vi "Host Error log.vi"(6 "Operation":enum16{"Create", "Write", "Close", "Header"}(ring)=enum."Write", 8 "error in":errorcluster, 11 "Enable":bool) -> (0 "error out":errorcluster, 2 "Error":string[][](array[string]))   [LabVIEW 2021]
uses:
  <vilib>/Utility/sysdir.llb/System Directory Type.ctl
  Main Engine/Controls/Main Engine Q Option.ctl
panel:
  in  "error in 2":errorcluster={"status"=TRUE, "code"=1, "source"="Dequeue Element in Host Error log.vi->MATSYA GUI.vi"}
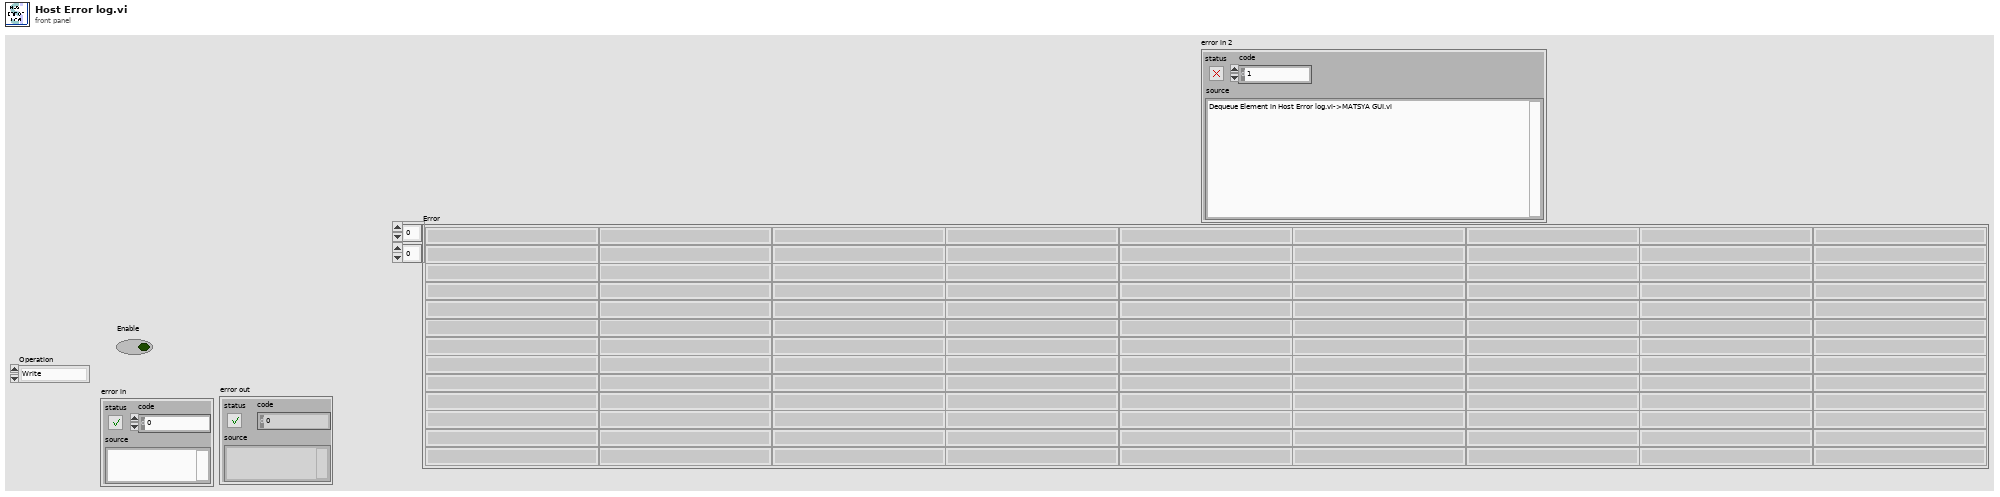
[diagram p1: front panel]
types:
  T1 = enum16{"open", "replace", "create", "open or create", "replace or create", "replace or create with confirmation"}
  T2 = typedef "Main Engine Q Option.ctl" = enum16{"Init", "Get"}
  T3 = typedef "System Directory Type.ctl" = i32
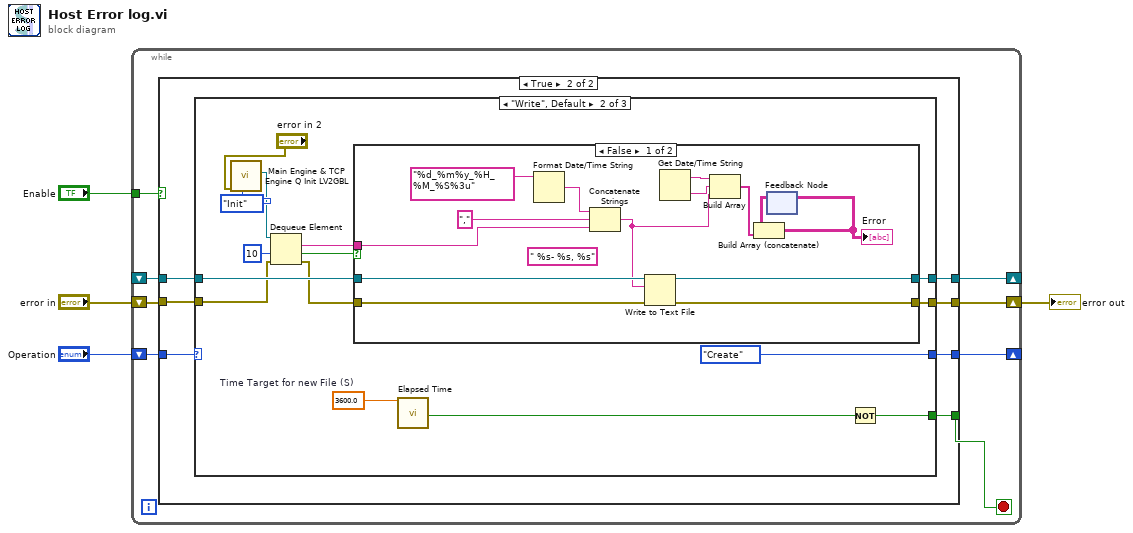
[diagram p0: block diagram]
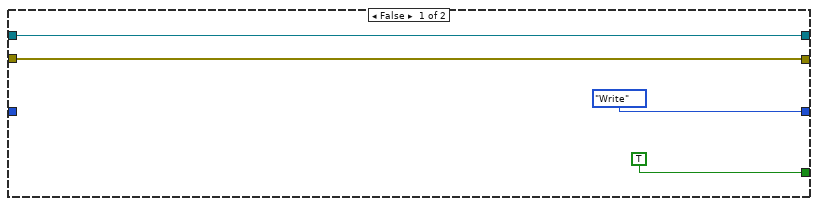
[diagram p2: hidden frame]
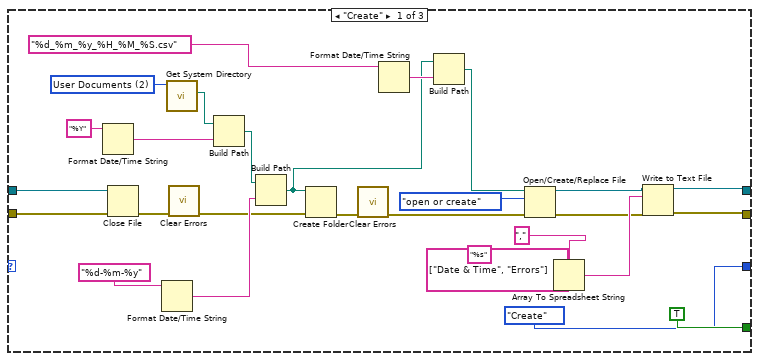
[diagram p3: hidden frame]
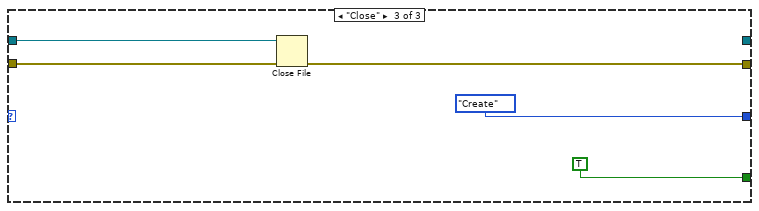
[diagram p5: hidden frame]
diagram:
  n1 = while {
    shift-right: [w11] -> _
    shift-left: _ -> [w10]
    shift-right: [w9] -> w2
    shift-left: "error in" -> [w8]
    tunnel: "Enable" -> [w7]
    shift-right: [w5] -> _
    shift-left: "Operation" -> [w12]
    stop <- w6 stop-if-true
    n2 = case shown="True" w7 {
      tunnel: w12 -> [_ w23]
      tunnel: [w16 w22] -> w11
      tunnel: w10 -> [w16 w21]
      tunnel: [w15 w20] -> w9
      tunnel: w8 -> [w15 w19]
      tunnel: [TRUE w18] -> w6
      tunnel: [enum16{"Create", "Write", "Close"}."Write" ("Operation 2") w17] -> w5
      frame False {
      }
      frame True {
        n3 = case shown="\"Write\", Default" w23 {
          tunnel: [w24 w64 _] -> w22
          tunnel: w21 -> [w34 w66 w85]
          tunnel: [w26 w65 w86] -> w20
          tunnel: w19 -> [w36 w54 w87]
          tunnel: [TRUE w62 TRUE] -> w18
          tunnel: [enum16{"Create", "Write", "Close", "Header"}."Create" ("Operation") enum16{"Create", "Write", "Close", "Header"}."Create" ("Operation") enum16{"Create", "Write", "Close", "Header"}."Create" ("Operation")] -> w17
          frame "Create" {
            w51 = T3 2 items=["User Home"=0, "User Desktop"=1, "User Documents"=2, "User Application Data"=3, "User Preferences"=4, "User Temporary"=5, "Public Documents"=6, "Public Application Data"=7, "Public Preferences"=8, "Public Cache"=13, "System Core Libraries"=9, "System Installed Libraries"=10, "Application Files"=11, "Boot Volume Root"=12] ("system directory type")
            n4 = Format Date/Time String(time format string (%c)="%Y") -> (date/time string=w47:string)  [unwired: 2 in]
            n5 = Close File(refnum=w34, error in=w36) -> (error out=w35:errorcluster)  [unwired: 1 out]
            n6 = Format Date/Time String(time format string (%c)="%d-%m-%y") -> (date/time string=w45:string)  [unwired: 2 in]
            n7 = call <vilib>:"Get System Directory.vi"("system directory type"=w51) -> ("system directory"=w48:path)  [unwired: 10 in]
            n8 = call <vilib>:"Clear Errors.vi"("error in (no error)"=w35) -> ("error out"=w33:errorcluster)  [unwired: 5 in, 1 out]
            n9 = Build Path(base path=w48, name or relative path=w47) -> (appended path=w46:path)
            n10 = Build Path(base path=w46, name or relative path=w45) -> (appended path=w38:path)
            n11 = Create Folder(path (use dialog)=w38, error in=w33) -> (error out=w40:errorcluster)  [unwired: 1 in, 2 out]
            n12 = call <vilib>:"Clear Errors.vi"("error in (no error)"=w40) -> ("error out"=w39:errorcluster)  [unwired: 5 in, 1 out]
            n13 = Format Date/Time String(time format string (%c)="%d_%m_%y_%H_%M_%S.csv") -> (date/time string=w43:string)  [unwired: 2 in]
            n14 = Build Path(base path=w38, name or relative path=w43) -> (appended path=w41:path)
            n15 = Open/Create/Replace File(file path (use dialog)=w41, error in=w39, operation (0:open)=T1."open or create") -> (refnum out=w25:refnum<file>, error out=w27:errorcluster)  [unwired: 3 in, 1 out]
            n16 = Array To Spreadsheet String(delimiter (Tab)=",", array=string[] ["Date & Time", "Errors"], 3:"%s" ("format string")) -> (spreadsheet string=w31:string)
            n17 = Write to Text File(file (use dialog)=w25, text=w31, error in=w27) -> (refnum out=w24:refnum<file>, error out=w26:errorcluster)  [unwired: 1 in, 1 out]
          }
          frame "Write", Default {
            w61 = 3600.0  # Time Target for new File (S)
            n18 = call "Main Engine & TCP Engine Q Init LV2GBL.vi"("Q Option"=Main_Engine_Q_Option."Init", "error in"="error in 2") -> ("TCP Enigine Q"=w52:refnum<queue>)  [unwired: 7 in, 2 out]
            n19 = Dequeue Element(queue=w52, timeout in ms (-1)=10, error in (no error)=w54) -> (element=w55:string, timed out?=w59:bool, error out=w60:errorcluster)  [unwired: 1 out]
            n20 = case shown="False" w59 {
              tunnel: w66 -> [w77 w82]
              tunnel: [w76 w81] -> w65
              tunnel: [w75 w82] -> w64
              tunnel: w60 -> [w74 w81]
              tunnel: w55 -> [w73 _]
              frame False {
                (unwired) " %s- %s, %s" ("format string")
                n21 = Format Date/Time String(time format string (%c)="%d_%m%y_%H_%M_%S%3u") -> (date/time string=w80:string)  [unwired: 2 in]
                n22 = Concatenate Strings(w80, "," ("delimiter (Tab)"), w73) -> (w67:string)
                n23 = Write to Text File(file (use dialog)=w77, text=w67, error in=w74) -> (refnum out=w75:refnum<file>, error out=w76:errorcluster)  [unwired: 1 in, 1 out]
                n24 = Get Date/Time String() -> (date string=w72:string, time string=w71:string)  [unwired: 3 in]
                n25 = Build Array(w72, w71, w67) -> (w70:string[])
                n26 = feedback #1() -> (w68:string[][])  [unwired: 1 in]
                n27 = Build Array (concatenate)(w68, w70) -> (w69:string[][])
                "Error" <- w69
                n28 = feedback-in #1(w69) -> ()
              }
              frame True {
              }
            }
            n29 = call "Elapsed Time"("Time Target (s)"=w61) -> ("Time has Elapsed"=w63:bool)  [unwired: 11 in, 7 out]
            n30 = Not(x=w63) -> (.not. x?=w62:bool)
          }
          frame "Close" {
            n31 = Close File(refnum=w85, error in=w87) -> (error out=w86:errorcluster)  [unwired: 1 out]
          }
        }
      }
    }
  }
  "error out" <- w2
